vi "Library Toolkit Path.vi"(7 "toolkit directory (none)":string, 11 "sub path of toolkit (none)":path) -> (8 "absolute toolkit path":path)   [LabVIEW 2012]
doc: "Returns a path inside some toolkit under the distribution root when in development mode or when this VI is not built into an executable. Otherwise, return the application executable path.\n\nThe purpose is to help locate dynamically loaded VIs by constructing a path relative to a single known location, which is the location of this VI. To work properly, this VI must therefore be located two deep under the distribution root or inside the built application executable.\n\nNormally, all VIs are built into one executable. The reason for allowing this VI to not be built into an executable even when not running under the development environment is that one can build an executable that dynamically loads as much as possible. In such a case, a minimal executable is built that dynamically loads the remainder of the VIs from the development source tree. This makes it easy to replace VIs without having to rebuild an executable."
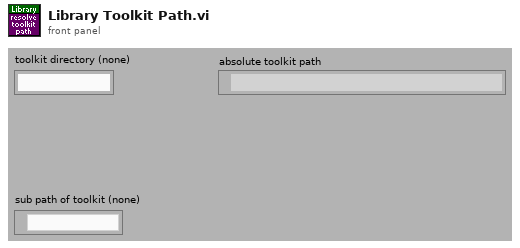
[diagram p1: front panel]
types:
  T1 = enum32{"invalid app kind", "Development System", "Run Time System", "Student Edition", "Embedded LabVIEW", "Evaluation", "Custom"}
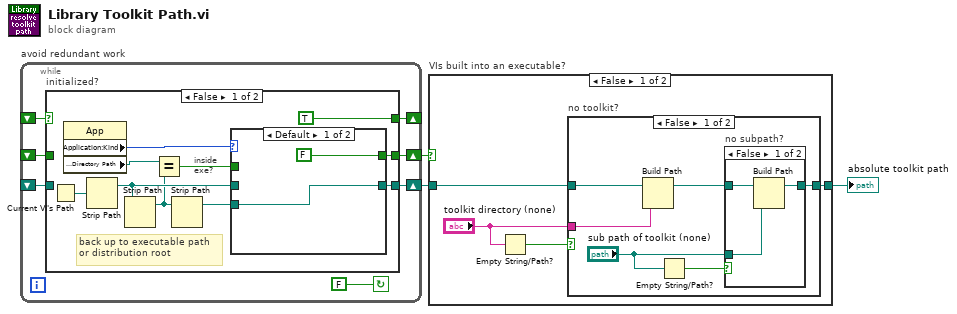
[diagram p0: block diagram]
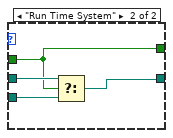
[diagram p5: hidden frame]
diagram:
  n1 = while "avoid redundant work" {
    shift-right: [w6] -> _
    shift-left: _ -> [w7]
    shift-right: [w9] -> w2
    shift-left: _ -> [w8]
    shift-right: [w5] -> w3
    shift-left: _ -> [w4]
    stop <- FALSE continue-if-true
    n2 = case "initialized?" shown="False" w7 {
      selector: w7 -> [_ w28]
      tunnel: [w20 w29] -> w9
      tunnel: w8 -> [_ w29]
      tunnel: [TRUE w28] -> w6
      tunnel: [w16 w27] -> w5
      tunnel: w4 -> [_ w27]
      frame False {
        # "inside\nexe?"
        # "back up to executable path\nor distribution root"
        n3 = Current VI's Path() -> (path=w17:path)
        n4 = property class="App"() -> ("Application:Kind"=w19:T1, "Application:Directory Path"=w13:path)  [unwired: 2 in, 2 out]
        n5 = Strip Path(path=w17) -> (stripped path=w15:path)  [unwired: 1 out]
        n6 = Strip Path(path=w15) -> (stripped path=w12:path)  [unwired: 1 out]
        n7 = Equal?(x=w13, y=w12) -> (x = y?=w11:bool)
        n8 = Strip Path(path=w12) -> (stripped path=w14:path)  [unwired: 1 out]
        n9 = case shown="Default" w19 {
          tunnel: [w21 w23] -> w20
          tunnel: w15 -> [_ w26]
          tunnel: [FALSE w25] -> w16
          tunnel: w14 -> [w21 w24]
          tunnel: w11 -> [_ w25]
          frame Default {
          }
          frame "Run Time System" {
            n10 = Select(t=w26, s=w25, f=w24) -> (s? t:f=w23:path)
          }
        }
      }
      frame True {
      }
    }
  }
  n11 = case "VIs built into an executable?" shown="False" w3 {
    tunnel: w2 -> [w32 w45]
    tunnel: [w30 w45] -> w1
    frame False {
      n12 = Empty String/Path?(string/path="toolkit directory (none)") -> (empty?=w33:bool)
      n13 = case "no toolkit?" shown="False" w33 {
        tunnel: w32 -> [w39 w44]
        tunnel: "toolkit directory (none)" -> [w38 _]
        tunnel: [w34 w44] -> w30
        frame False {
          n14 = Build Path(base path=w39, name or relative path=w38) -> (appended path=w37:path)
          n15 = Empty String/Path?(string/path="sub path of toolkit (none)") -> (empty?=w35:bool)
          n16 = case "no subpath?" shown="False" w35 {
            tunnel: w37 -> [w42 w43]
            tunnel: "sub path of toolkit (none)" -> [w41 _]
            tunnel: [w40 w43] -> w34
            frame False {
              n17 = Build Path(base path=w42, name or relative path=w41) -> (appended path=w40:path)
            }
            frame True {
            }
          }
        }
        frame True {
        }
      }
    }
    frame True {
    }
  }
  "absolute toolkit path" <- w1
